vi "ModbusPort.vi"(10 "ModbusPortSettings":T1={"TxPort"="ModbusPort1Tx", "TxDataFIFO"="ModbusPort1TxFIFO", "TxInternalDataFIFO"="ModbusPort1TxInternalFIFO", "TxHealthAndStatusFIFO"="ModbusPort1TxHealthAndStatusFIFO", "RxPort"="ModbusPort1Rx", "RxDataFIFO"="ModbusPort1RxFIFO", "RxHealthAndStatusFIFO"="ModbusPort1RxHealthAndStatusFIFO", "BaseHealthAndStatusAddress"=0, "WaitForRxFrameRegister"="ModbusPort1WaitForRxControl", "IRQAddress"=0, "TriggerIRQRegister"="ModbusPort1IRQControl", "InternalHealthAndStatusFIFO"="InternalHealthAndStatusFIFO", "SoftwareControlledTrigger"="ModbusSoftwareControlledTrigger"}) -> ()   [LabVIEW 2016, in "FPGAModbus.lvlib"]
uses:
  FPGAModbus.lvlib
  DataTypes/ModbusPortSettings.ctl
  <vilib>/rvi/eio/common/nirviEmuTemplateMethod_errors.vi
  <vilib>/rvi/Emulation/niFpgaProcessEmulError.vi
  <vilib>/eio/EIONode/EIONode.xnode
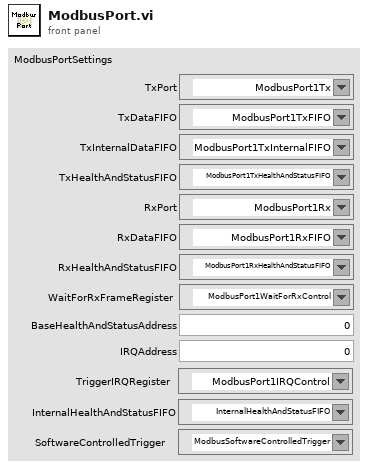
[diagram p1: front panel]
types:
  T1 = typedef "FPGAModbus.lvlib/ModbusPortSettings.ctl" = cluster{"TxPort":refnum<k21>, "TxDataFIFO":refnum<k21>, "TxInternalDataFIFO":refnum<k21>, "TxHealthAndStatusFIFO":refnum<k21>, "RxPort":refnum<k21>, "RxDataFIFO":refnum<k21>, "RxHealthAndStatusFIFO":refnum<k21>, "BaseHealthAndStatusAddress":u32, "WaitForRxFrameRegister":refnum<k21>, "IRQAddress":u8, "TriggerIRQRegister":refnum<k21>, "InternalHealthAndStatusFIFO":refnum<k21>, "SoftwareControlledTrigger":refnum<k21>}
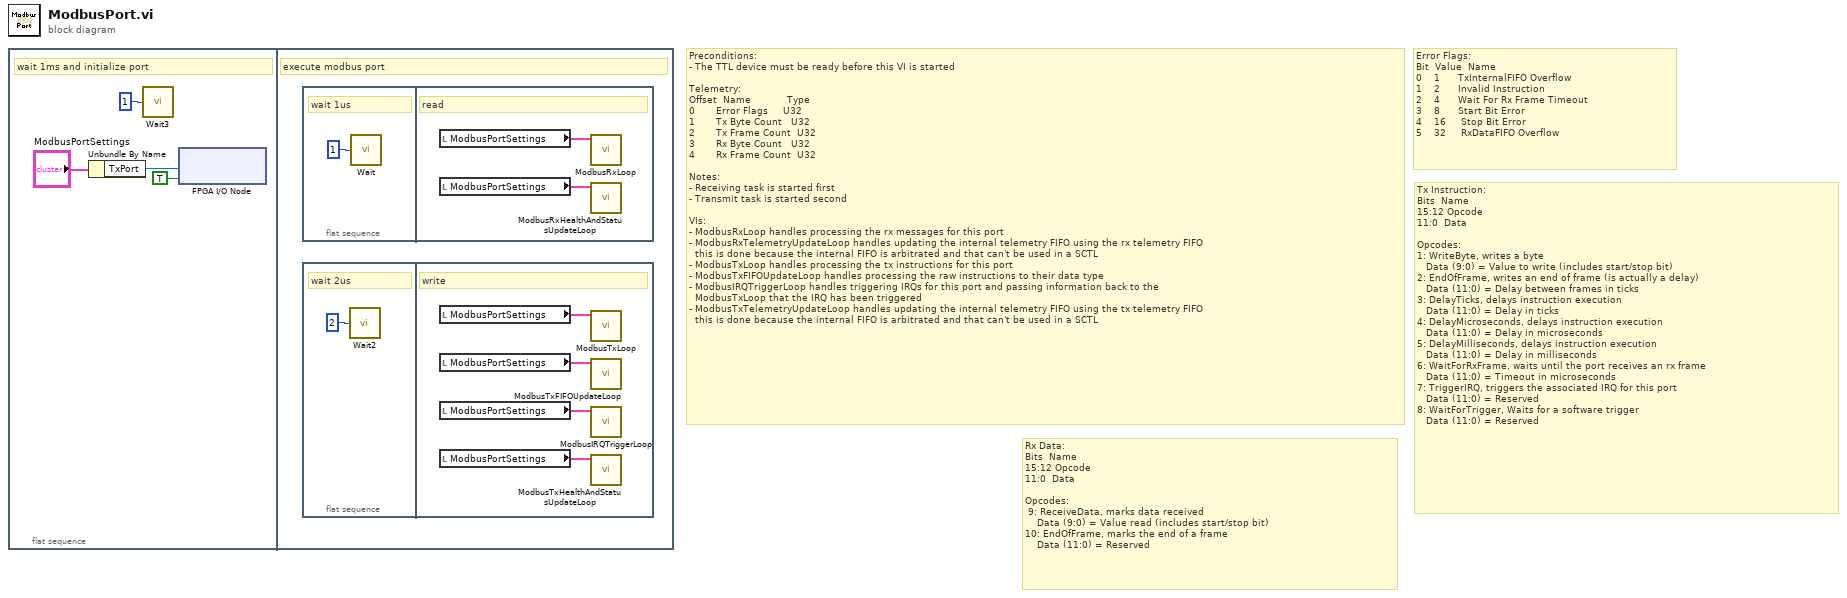
[diagram p0: block diagram]
diagram:
  # "Rx Data:\nBits  Name\n15:12 Opcode\n11:0  Data\n\nOpcodes:\n 9: ReceiveData, marks data received\n    Data (9:0) = Value read (includes start/stop bit)\n10: EndOfFrame, marks the end of a frame\n    Data (11:0) = Reserved"
  # "Tx Instruction:\nBits  Name\n15:12 Opcode\n11:0  Data\n\nOpcodes:\n1: WriteByte, writes a byte\n   Data (9:0) = Value to write (includes start/stop bit)\n2: EndOfFrame, writes an end of frame (is actually a delay)\n   Data (11:0) = Delay between frames in ticks\n3: DelayTicks, delays instruction execution\n   Data (11:0) = Delay in ticks\n4: DelayMicroseconds, delays instruction execution\n   Data (11:0) = Delay in microseconds\n5: DelayMilliseconds, delays instruction execution\n   Data (11:0) = Delay in milliseconds\n6: WaitForRxFrame, waits until the port receives an rx frame\n   Data (11:0) = Timeout in microseconds\n7: TriggerIRQ, triggers the associated IRQ for this port\n   Data (11:0) = Reserved\n8: WaitForTrigger, Waits for a software trigger\n   Data (11:0) = Reserved"
  # "Error Flags:\nBit  Value  Name\n0    1      TxInternalFIFO Overflow\n1    2      Invalid Instruction \n2    4      Wait For Rx Frame Timeout\n3    8      Start Bit Error\n4    16     Stop Bit Error\n5    32     RxDataFIFO Overflow"
  # "Preconditions:\n- The TTL device must be ready before this VI is started\n\nTelemetry:\nOffset  Name            Type\n0       Error Flags     U32         \n1       Tx Byte Count   U32\n2       Tx Frame Count  U32\n3       Rx Byte Count   U32\n4       Rx Frame Count  U32\n\nNotes:\n- Receiving task is started first\n- Transmit task is started second\n\nVIs:\n- ModbusRxLoop handles processing the rx messages for this port\n- ModbusRxTelemetryUpdateLoop handles updating the internal telemetry FIFO using the rx telemetry FIFO\n  this is done because the internal FIFO is arbitrated and that can't be used in a SCTL\n- ModbusTxLoop handles processing the tx instructions for this port\n- ModbusTxFIFOUpdateLoop handles processing the raw instructions to their data type\n- ModbusIRQTriggerLoop handles triggering IRQs for this port and passing information back to the\n  ModbusTxLoop that the IRQ has been triggered\n- ModbusTxTelemetryUpdateLoop handles updating the internal telemetry FIFO using the tx telemetry FIFO\n  this is done because the internal FIFO is arbitrated and that can't be used in a SCTL"
  n1 = flat-sequence {
    frame #0 {
      # "wait 1ms and initialize port"
      n2 = Unbundle By Name("ModbusPortSettings") -> ("TxPort"=w2:refnum<k21>)
      n3 = call "Wait3"("Count(mSec)"=u32 1 ("Count(Ticks)")) -> ()  [unwired: 1 out]
      n4 = xnode "FPGA I/O Node"("I/O Item"=TRUE, "FPGA I/O In"=w2) -> ()  [unwired: 1 out]
    }
    frame #1 {
      # "execute modbus port"
      n5 = flat-sequence {
        frame #0 {
          # "wait 1us"
          n6 = call "Wait"("Count(uSec)"=u32 1 ("Count(Ticks)")) -> ()  [unwired: 1 out]
        }
        frame #1 {
          # "read"
          n7 = local read "ModbusPortSettings"() -> (w12:T1)
          n8 = local read "ModbusPortSettings"() -> (w11:T1)
          n9 = call "ModbusRxLoop.vi"("ModbusPortSettings"=w12) -> ()  [unwired: 11 in]
          n10 = call "ModbusRxHealthAndStatusUpdateLoop.vi"("ModbusPortSettings"=w11) -> ()  [unwired: 11 in]
        }
      }
      n11 = flat-sequence {
        frame #0 {
          # "wait 2us"
          n12 = call "Wait2"("Count(uSec)"=u32 2 ("Count(Ticks)")) -> ()  [unwired: 1 out]
        }
        frame #1 {
          # "write"
          n13 = local read "ModbusPortSettings"() -> (w9:T1)
          n14 = local read "ModbusPortSettings"() -> (w8:T1)
          n15 = local read "ModbusPortSettings"() -> (w7:T1)
          n16 = local read "ModbusPortSettings"() -> (w6:T1)
          n17 = call "ModbusTxLoop.vi"("ModbusPortSettings"=w9) -> ()  [unwired: 11 in]
          n18 = call "ModbusTxFIFOUpdateLoop.vi"("Modbus Port Settings"=w8) -> ()  [unwired: 11 in]
          n19 = call "ModbusIRQTriggerLoop.vi"("ModbusPortSettings"=w7) -> ()  [unwired: 11 in]
          n20 = call "ModbusTxHealthAndStatusUpdateLoop.vi"("ModbusPortSettings"=w6) -> ()  [unwired: 11 in]
        }
      }
    }
  }
